vi "OSICS_Set_Power.vi"(7 "OSICS slot":i32=1 min=1 max=8 step=1, 8 "error in":errorcluster, 9 "P Value":dbl format="%.2g", 10 "Power Unit(False:dBm)":bool, 11 "VISA IN":refnum<visa-resource-name>) -> (0 "error out":errorcluster, 3 "VISA OUT":refnum<visa-resource-name>, 5 "ERR":i32)   [LabVIEW 2014, in "OSICS_LIB.lvlib"]
doc: "This Vi sets the power units and power output value of OSICS laser modules.\nModules: DFB, ECL, T100, TLS-50 and TLS-AG."
uses:
  OSICS_LIB.lvlib
panel:
  # "Basic Function to set the power units and power output\nfor the OSICS modules"
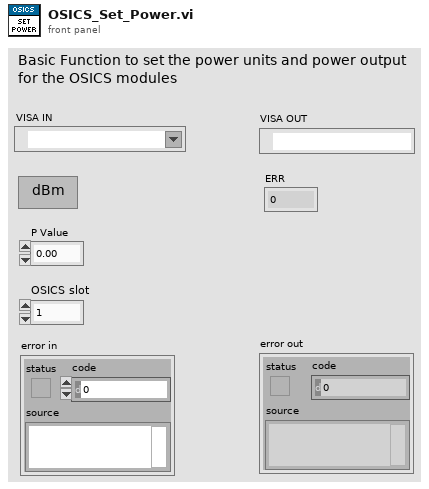
[diagram p1: front panel]
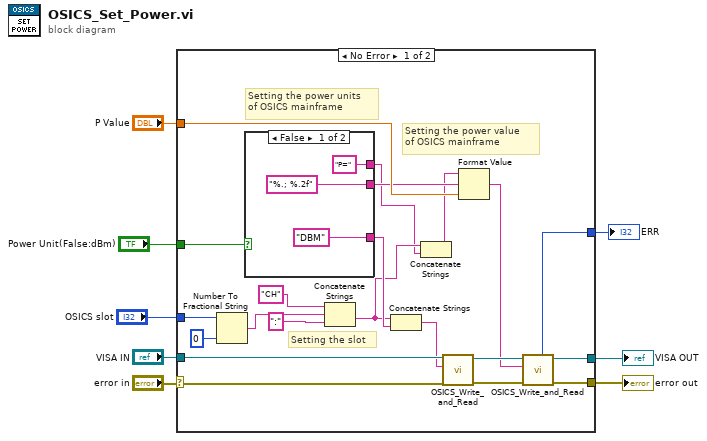
[diagram p0: block diagram]
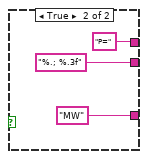
[diagram p2: hidden frame]
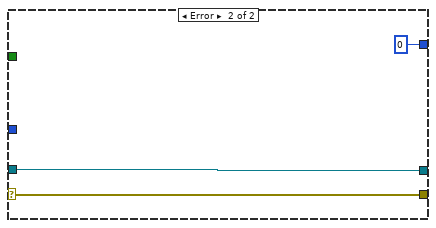
[diagram p3: hidden frame]
diagram:
  n1 = case shown="No Error" "error in" {
    selector: "error in" -> [w20 w37]
    tunnel: "Power Unit(False:dBm)" -> [w29 _]
    tunnel: "VISA IN" -> [w28 w38]
    tunnel: "P Value" -> [w25 _]
    tunnel: [w24 w38] -> w7
    tunnel: [w23 w37] -> w6
    tunnel: [w9 0 ("ERR")] -> w2
    tunnel: "OSICS slot" -> [w19 _]
    frame No Error {
      # "Setting the slot"
      # "Setting the power value\nof OSICS mainframe"
      # "Setting the power units\nof OSICS mainframe"
      n2 = Number To Fractional String(number=w19, precision (6)=i16 0) -> (F-format string=w16:string)  [unwired: 2 in]
      n3 = case shown="False" w29 {
        tunnel: ["DBM" "MW"] -> w13
        tunnel: ["%.; %.2f" ("format string") "%.; %.3f" ("format string")] -> w21
        tunnel: ["P=" "P="] -> w11
        frame False {
        }
        frame True {
        }
      }
      n4 = Concatenate Strings("CH" ("string"), w16, ":" ("string")) -> (w12:string)
      n5 = Concatenate Strings(w12, w13) -> (w14:string)
      n6 = Concatenate Strings(w12, w11) -> (w10:string)
      n7 = call "OSICS_Write_and_Read.vi"("error in (no error)"=w20, "String to Send"=w14, "VISA IN"=w28) -> ("error out"=w26:errorcluster, "VISA OUT"=w27:refnum<visa-resource-name>)  [unwired: 5 in, 2 out]
      n8 = Format Value(string ("")=w10, format string=w21, value (0)=w25) -> (output string=w22:string)
      n9 = call "OSICS_Write_and_Read.vi"("error in (no error)"=w26, "String to Send"=w22, "VISA IN"=w27) -> ("error out"=w23:errorcluster, "VISA OUT"=w24:refnum<visa-resource-name>, "ERR"=w9:i32)  [unwired: 5 in, 1 out]
    }
    frame Error {
    }
  }
  "error out" <- w6
  "VISA OUT" <- w7
  "ERR" <- w2
